vi "sv_Continuous Swept-Sine Errors.vi"(11 "continuous swept-sine error":T1) -> (0 "error out":errorcluster)   [LabVIEW 2017, in "SoundVib_ContSweptSine.lvlib"]
uses:
  <vilib>/addons/Sound and Vibration/svt_Continuous Swept Sine/SoundVib_ContSweptSine.lvlib
  <vilib>/addons/Sound and Vibration/svt_Continuous Swept Sine/subVIs/sv_Continuous Swept-Sine Errors.ctl
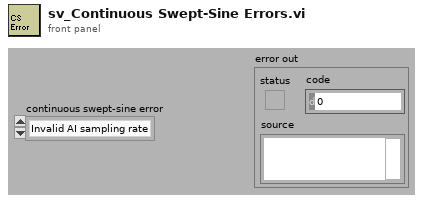
[diagram p1: front panel]
types:
  T1 = typedef "SoundVib_ContSweptSine.lvlib/sv_Continuous Swept-Sine Errors.ctl" = enum16{"Invalid AI sampling rate", "Item not found", "Invalid initial phase"}
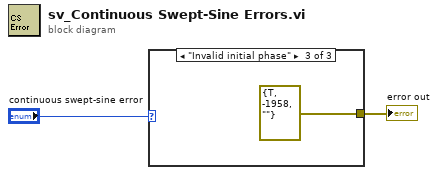
[diagram p0: block diagram]
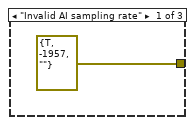
[diagram p2: hidden frame]
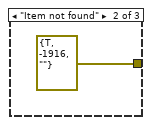
[diagram p3: hidden frame]
diagram:
  n1 = case shown="\"Invalid initial phase\"" "continuous swept-sine error" {
    tunnel: [errorcluster {"status"=TRUE, "code"=-1957, "source"=""} ("error in (no error)") errorcluster {"status"=TRUE, "code"=-1916, "source"=""} ("error in (no error)") errorcluster {"status"=TRUE, "code"=-1958, "source"=""} ("error in (no error)")] -> w1
    frame "Invalid AI sampling rate" {
    }
    frame "Item not found" {
    }
    frame "Invalid initial phase" {
    }
  }
  "error out" <- w1
